vi "camera-startup.vi"() -> ()   [LabVIEW 2014]
uses:
  SubVIs/Initilize Globals.vi
  lib/Andorlib/atmcd32d.lvlib
panel:
  in  "Cooling":bool
  in  "Warm up CCD & Turn Off Camera":bool
  out "Cooling Status":T1
  out "Detector Temperature":i32(graph)
  out "Camera Properties":T2
  in  "Temp. Set Point":dbl(slide) scale=-120.0..20.0 scale format="%_1f"
  out "Status":string
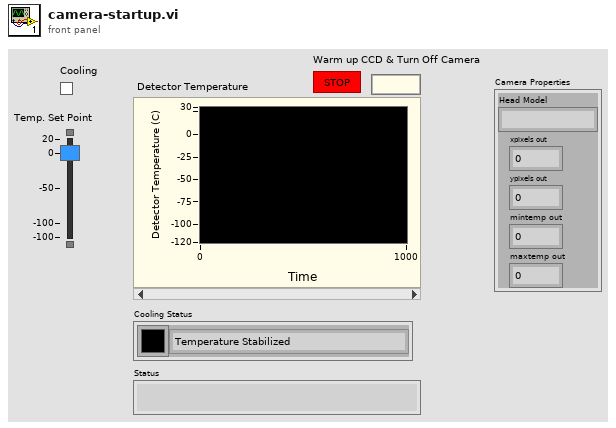
[diagram p1: front panel]
types:
  T1 = cluster{"Cooling Status":enum16{"Temperature Stabilized", "Waiting to Stabilize Temperature", "Cooling is Turned Off", "Have not yet Reached Set Temperature"}, "Color Box":u32}
  T2 = cluster{"Head Model":string, "xpixels out":i32, "ypixels out":i32, "mintemp out":i32, "maxtemp out":i32}
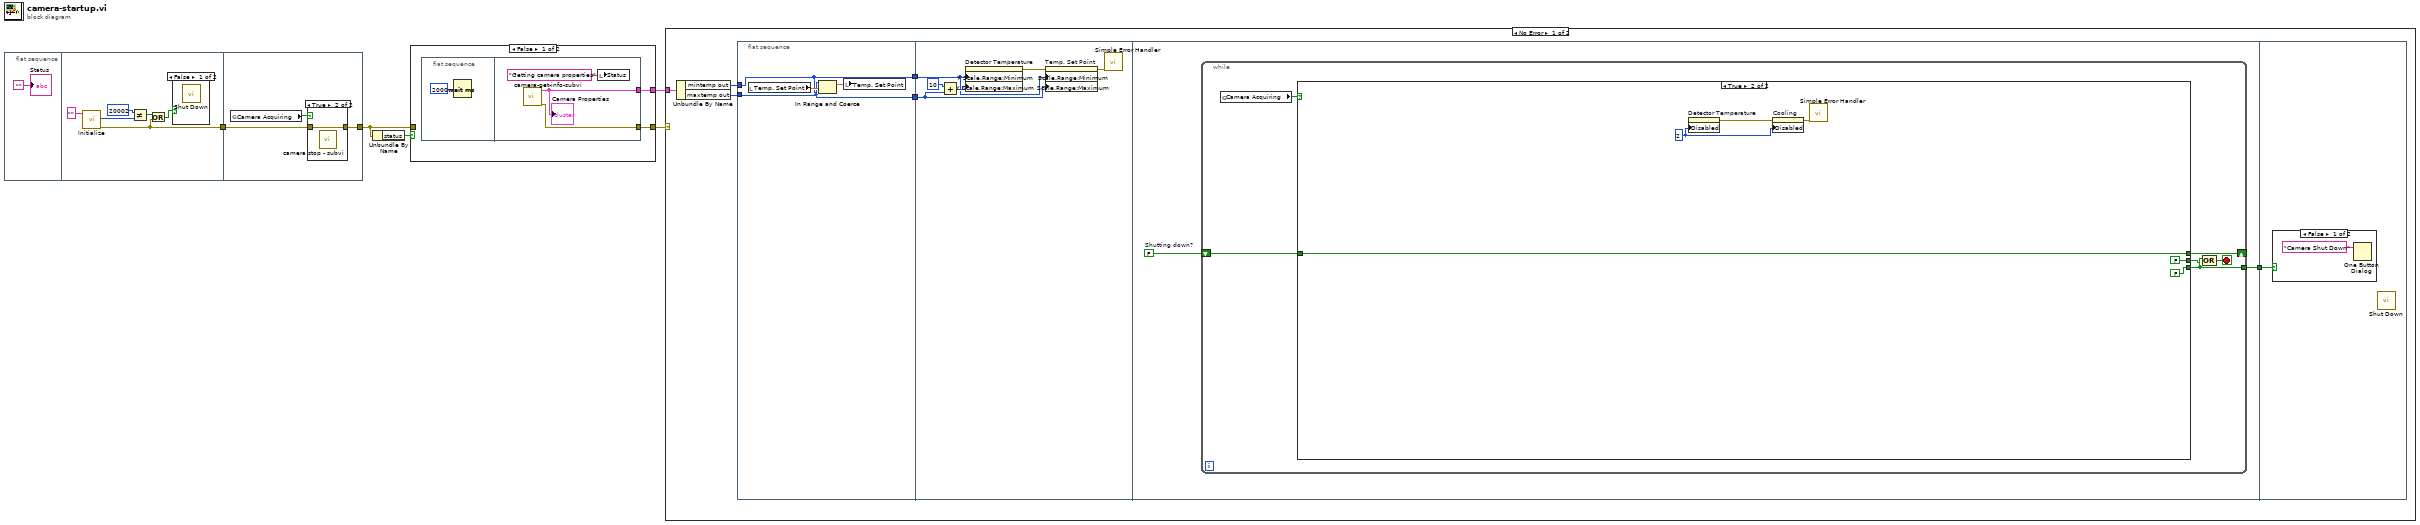
[diagram p0: block diagram]
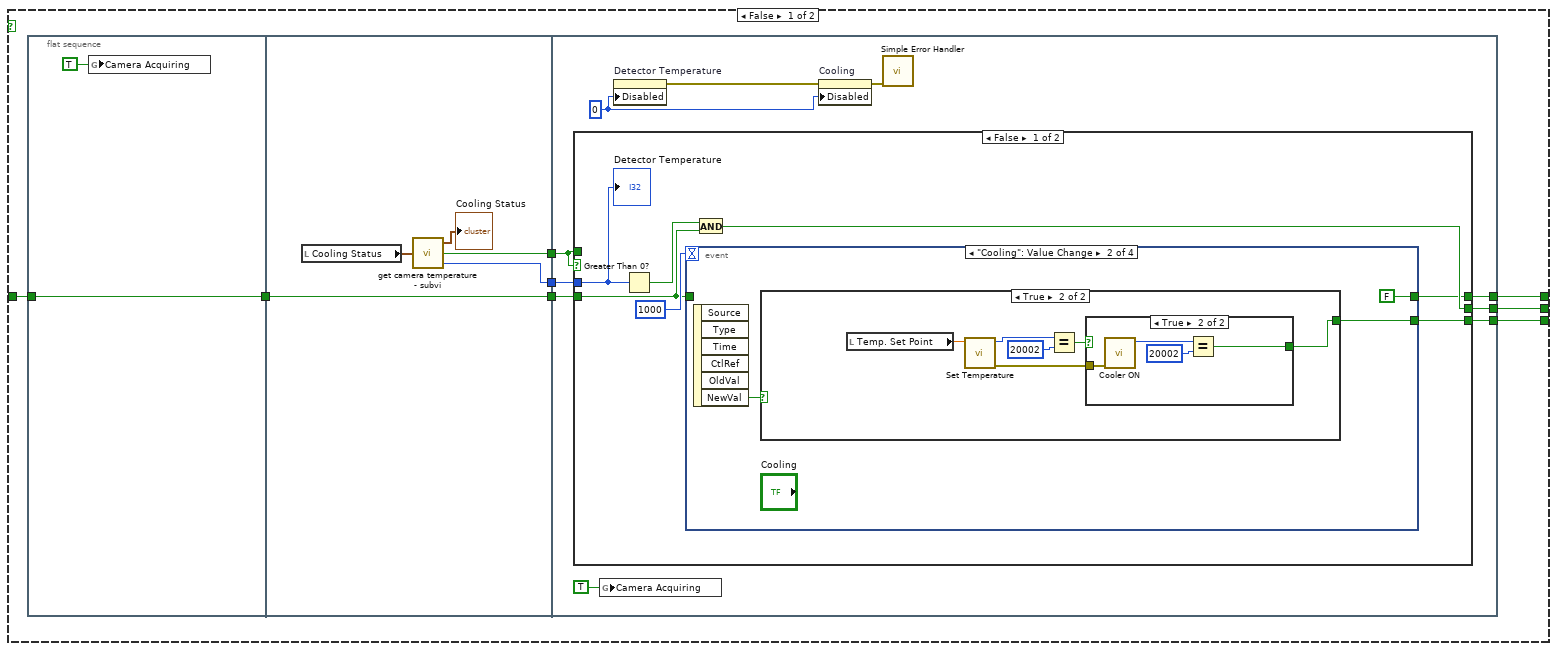
[diagram p2: hidden frame]
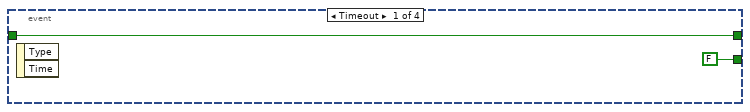
[diagram p3: hidden frame]
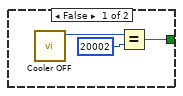
[diagram p4: hidden frame]
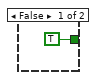
[diagram p5: hidden frame]
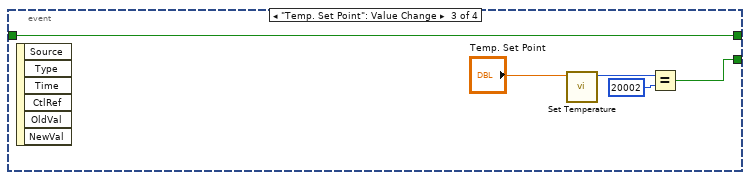
[diagram p6: hidden frame]
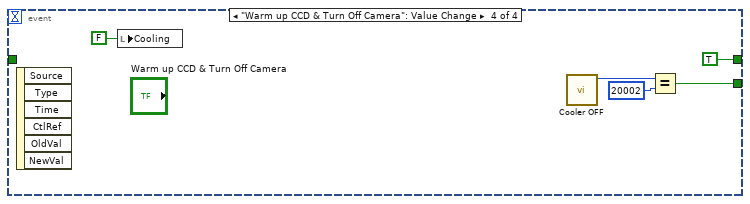
[diagram p7: hidden frame]
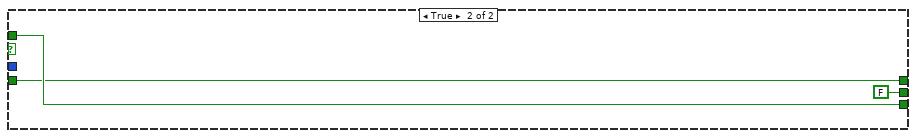
[diagram p8: hidden frame]
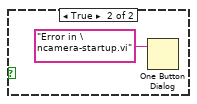
[diagram p9: hidden frame]
diagram:
  n1 = flat-sequence {
    tunnel: [w10] -> w5
    tunnel: w5 -> [w14]
    tunnel: [w13] -> w3
    frame #0 {
      "Status" <- ""
    }
    frame #1 {
      n2 = call "Initialize.vi"("dir"="") -> ("error out"=w10:errorcluster, "function return"=w8:u32)  [unwired: 8 in, 1 out]
      n3 = Not Equal?(x=u32 20002, y=w8) -> (x != y?=w9:bool)
      n4 = Or(x=w9, y=w10) -> (x .or. y?=w11:bool)
      n5 = case shown="False" w11 {
        frame False {
          n6 = call "Shut Down.vi"() -> ()  [unwired: 10 in, 2 out]
        }
        frame True {
        }
      }
    }
    frame #2 {
      n7 = global read "Initilize Globals.vi" "Camera Acquiring"() -> (w15:bool)
      n8 = case shown="True" w15 {
        tunnel: [w16 w17] -> w13
        tunnel: w14 -> [w16 w17]
        frame False {
        }
        frame True {
          n9 = call "camera stop - subvi.vi"() -> ()  [unwired: 1 in]
        }
      }
    }
  }
  n10 = Unbundle By Name(w3) -> ("status"=w4:bool)
  n11 = case shown="False" w4 {
    tunnel: w3 -> [_ w24]
    tunnel: [w19 w24] -> w2
    tunnel: [w18 _] -> w1
    frame False {
      n12 = flat-sequence {
        tunnel: [w22] -> w19
        tunnel: [w21] -> w18
        frame #0 {
          n13 = Wait (ms)(milliseconds to wait=u32 2000) -> ()  [unwired: 1 out]
        }
        frame #1 {
          n14 = call "camera-get-info-subvi.vi"() -> ("error out"=w22:errorcluster, "Camera Properties"=w21:T2)  [unwired: 10 in]
          "Camera Properties" <- w21
          n15 = local write "Status"("Getting camera properties" ("Status")) -> ()
        }
      }
    }
    frame True {
    }
  }
  n16 = case shown="No Error" w2 {
    tunnel: w1 -> [w30 _]
    frame No Error {
      n17 = Unbundle By Name(w30) -> ("mintemp out"=w29:i32, "maxtemp out"=w28:i32)
      n18 = flat-sequence {
        tunnel: w29 -> [w31]
        tunnel: w28 -> [w32]
        tunnel: [w32] -> w27
        tunnel: [w31] -> w26
        tunnel: w27 -> [w37]
        tunnel: w26 -> [w38]
        tunnel: [w41] -> w25
        tunnel: w25 -> [w119]
        frame #0 {
          n19 = local read "Temp. Set Point"() -> (w34:dbl)
          n20 = In Range and Coerce(upper limit=w32, x=w34, lower limit=w31) -> (coerced(x)=w33:dbl)  [unwired: 1 out]
          n21 = local write "Temp. Set Point"(w33) -> ()
        }
        frame #1 {
          n22 = Add(x=10, y=w37) -> (x+y=w39:i32)
          n23 = property on="Detector Temperature" class="WFChart (strict)"("Y Scale.Range:Minimum"=w38, "Y Scale.Range:Maximum"=w39) -> (error out=w35:errorcluster)  [unwired: 2 in, 1 out]
          n24 = property on="Temp. Set Point" class="Slide (strict)"(error in=w35, "Scale.Range:Minimum"=w38, "Scale.Range:Maximum"=w37) -> (error out=w36:errorcluster)  [unwired: 1 in, 1 out]
          n25 = call <vilib>:"Simple Error Handler.vi"("error in (no error)"=w36) -> ()  [unwired: 1 in, 8 out]
        }
        frame #2 {
          w42 = FALSE  # Shutting down?
          n26 = while {
            shift-right: [w46] -> _
            shift-left: w42 -> [w47]
            tunnel: [w45] -> w41
            stop <- w44 stop-if-true
            n27 = global read "Initilize Globals.vi" "Camera Acquiring"() -> (w48:bool)
            n28 = case shown="True" w48 {
              tunnel: w47 -> [w52 w117]
              tunnel: [w54 FALSE] -> w43
              tunnel: [w49 w117] -> w46
              tunnel: [w50 FALSE] -> w45
              frame False {
                n29 = flat-sequence {
                  tunnel: [w57] -> w53
                  tunnel: w52 -> [w57]
                  tunnel: [w61] -> w56
                  tunnel: [w60] -> w55
                  tunnel: w53 -> [w59]
                  tunnel: [w59] -> w51
                  tunnel: w55 -> [w72]
                  tunnel: w56 -> [w71]
                  tunnel: [w70] -> w54
                  tunnel: w51 -> [w69]
                  tunnel: [w65] -> w50
                  tunnel: [w64] -> w49
                  frame #0 {
                    n30 = global write "Initilize Globals.vi" "Camera Acquiring"(TRUE) -> ()
                  }
                  frame #1 {
                    n31 = local read "Cooling Status"() -> (w63:T1)
                    n32 = call "get camera temperature - subvi.vi"("Cooling Status In"=w63) -> ("Cooling Status Out"=→"Cooling Status":T1, "Error?"=w60:bool, "temperature out"=w61:i32)
                  }
                  frame #2 {
                    w68 = u8 0 ("Disabled")
                    n33 = case shown="False" w72 {
                      tunnel: w72 -> [_ w112]
                      tunnel: w71 -> [w79 _]
                      tunnel: [w75 w112] -> w65
                      tunnel: [w77 FALSE] -> w70
                      tunnel: w69 -> [w76 w110]
                      tunnel: [w74 w110] -> w64
                      frame False {
                        n34 = Greater Than 0?(x=w79) -> (x > 0?=w78:bool)
                        n35 = event shown="[1] \"Cooling\": Value Change" {
                          selector: _ -> [_ _ _ _]
                          dyn-events: _ -> [_ _ _ _]
                          timeout: 1000 -> [_ _ _ _]
                          tunnel: w76 -> [w82 _ w104 _]
                          tunnel: [w82 FALSE w104 TRUE] -> w74
                          tunnel: [FALSE ("status") w84 w100 w105] -> w75
                          event Timeout {
                            n36 = event-data() -> ()  [unwired: 3 out]
                          }
                          event "Cooling": Value Change {
                            n37 = event-data() -> ("NewVal"=w83:bool)  [unwired: 6 out]
                            n38 = case shown="True" w83 {
                              tunnel: [w87 w90] -> w84
                              frame False {
                                n39 = call "Cooler OFF.vi"() -> ("function return"=w86:u32)  [unwired: 10 in, 1 out]
                                n40 = Equal?(x=w86, y=20002) -> (x = y?=w87:bool)
                              }
                              frame True {
                                n41 = local read "Temp. Set Point"() -> (w94:dbl)
                                n42 = call "Set Temperature.vi"("temperature"=w94) -> ("error out"=w89:errorcluster, "function return"=w92:u32)  [unwired: 9 in]
                                n43 = Equal?(x=w92, y=20002) -> (x = y?=w93:bool)
                                n44 = case shown="True" w93 {
                                tunnel: [TRUE w96] -> w90
                                tunnel: w89 -> [_ w99]
                                frame False {
                                }
                                frame True {
                                n45 = call "Cooler ON.vi"("error in (no error)"=w99) -> ("function return"=w97:u32)  [unwired: 9 in, 1 out]
                                n46 = Equal?(x=w97, y=20002) -> (x = y?=w96:bool)
                                }
                                }
                              }
                            }
                          }
                          event "Temp. Set Point": Value Change {
                            n47 = event-data() -> ()  [unwired: 7 out]
                            n48 = call "Set Temperature.vi"("temperature"="Temp. Set Point") -> ("function return"=w101:u32)  [unwired: 9 in, 1 out]
                            n49 = Equal?(x=w101, y=20002) -> (x = y?=w100:bool)
                          }
                          event "Warm up CCD & Turn Off Camera": Value Change {
                            n50 = event-data() -> ()  [unwired: 7 out]
                            n51 = local write "Cooling"(FALSE ("Cooling")) -> ()
                            n52 = call "Cooler OFF.vi"() -> ("function return"=w106:u32)  [unwired: 10 in, 1 out]
                            n53 = Equal?(x=w106, y=20002) -> (x = y?=w105:bool)
                          }
                        }
                        n54 = And(x=w78, y=w76) -> (x .and. y?=w77:bool)
                        "Detector Temperature" <- w79
                      }
                      frame True {
                      }
                    }
                    n55 = global write "Initilize Globals.vi" "Camera Acquiring"(TRUE) -> ()
                    n56 = property on="Detector Temperature" class="WFChart (strict)"("Disabled"=w68) -> (error out=w67:errorcluster)  [unwired: 2 in, 1 out]
                    n57 = property on="Cooling" class="Bool (strict)"(error in=w67, "Disabled"=w68) -> (error out=w66:errorcluster)  [unwired: 1 in, 1 out]
                    n58 = call <vilib>:"Simple Error Handler.vi"("error in (no error)"=w66) -> ()  [unwired: 1 in, 8 out]
                  }
                }
              }
              frame True {
                w115 = u8 2 ("Disabled")
                n59 = property on="Detector Temperature" class="WFChart (strict)"("Disabled"=w115) -> (error out=w114:errorcluster)  [unwired: 2 in, 1 out]
                n60 = property on="Cooling" class="Bool (strict)"(error in=w114, "Disabled"=w115) -> (error out=w113:errorcluster)  [unwired: 1 in, 1 out]
                n61 = call <vilib>:"Simple Error Handler.vi"("error in (no error)"=w113) -> ()  [unwired: 1 in, 8 out]
              }
            }
            n62 = Compound Arithmetic op=OR(w45, w43) -> (w44:bool)
          }
        }
        frame #3 {
          n63 = case shown="False" w119 {
            frame False {
              n64 = One Button Dialog(message="Camera Shut Down" ("string")) -> ()  [unwired: 2 out]
            }
            frame True {
              n65 = One Button Dialog(message="Error in \ncamera-startup.vi" ("string")) -> ()  [unwired: 2 out]
            }
          }
          n66 = call "Shut Down.vi"() -> ()  [unwired: 10 in, 2 out]
        }
      }
    }
    frame Error {
    }
  }
